vi "TW Convert Top Level.vi"() -> ()   [LabVIEW 2021, in "Plugin Generator.lvlib"]
uses:
  Plugin Generator.lvlib
panel:
  out "error out":errorcluster
  in  "Text color":u32(colorbox)
  in  "Background":u32(colorbox)=14457856
  in  "New Name":string="CIFRocks"
  in  "Template Project Path":path=path "D:/dev/Plugins/ROCK - Copy/Tests/Template Interactive Test.lvproj"
  in  "Icon Text":string="RK-ON"
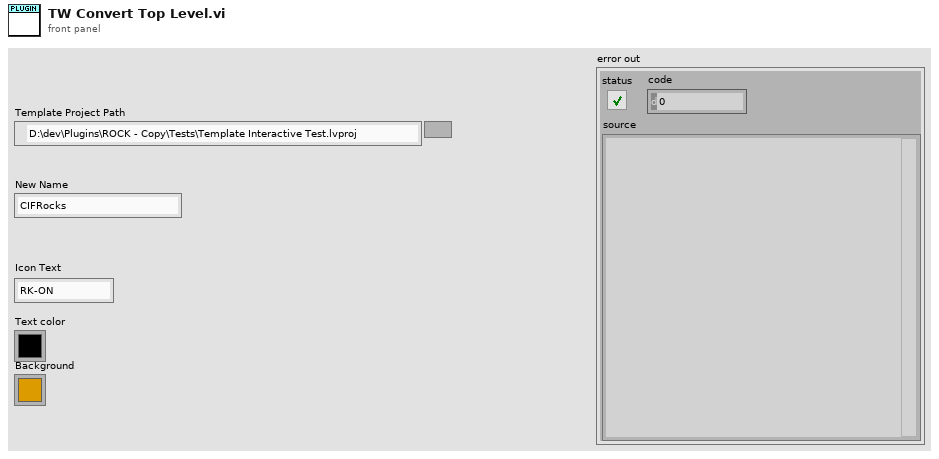
[diagram p1: front panel]
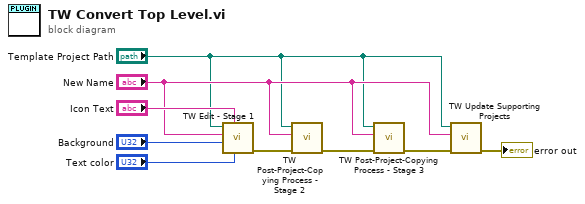
[diagram p0: block diagram]
diagram:
  n1 = call "TW Edit - Stage 1.vi"("Text color"="Text color", "Icon Text"="Icon Text", "Background"="Background", "New Subname"="New Name", "Template Project Path"="Template Project Path") -> ("error out"=w6:errorcluster)  [unwired: 5 in, 1 out]
  n2 = call "TW Post-Project-Copying Process - Stage 2.vi"("error in"=w6, "New Subname"="New Name", "Template Project Path"="Template Project Path") -> ("error out"=w5:errorcluster)  [unwired: 8 in]
  n3 = call "TW Post-Project-Copying Process - Stage 3.vi"("error in"=w5, "New Subname"="New Name", "Template Project Path"="Template Project Path") -> ("error out"=w4:errorcluster)  [unwired: 8 in]
  n4 = call "TW Update Supporting Projects.vi"("error in (no error)"=w4, "New Name"="New Name", "Template Project Path"="Template Project Path") -> ("error out"=→"error out":errorcluster)  [unwired: 8 in]
